vi "Init.vi"(4 "Virt Instrs":string="{\n\t\"Virt Instrs\": [\n\t\t{\"Target Ident\": \"Photosensor\",\"Instr Ident\": \"SimulatedScope\",\"Const Action Data\": \"0\",\"Class\": \"HAL GOOP4.lvlib:Virt Instr Base.lvclass\"},\n\t\t{\"Target Ident\": \"Powersensor\",\"Instr Ident\": \"SimulatedScope\",\"Const Action Data\": \"1\",\"Class\": \"Virt Instrs Scope.lvlib:Virt Voltage Reader.lvclass\"},\n\t\t{\"Target Ident\": \"Excitation\",\"Instr Ident\": \"SimulatedFGen\",\"Const Action Data\": \"0\",\"Class\": \"Virt Instrs FGen.lvlib:Virt Voltage Generator.lvclass\"}\n\t]\n}", 6 "Instr CFGs":string[](array[string]), 8 "error in (no error)":errorcluster, 11 "HAL GOOP4:Series Base in":refnum<class "Series Base.lvclass">) -> (0 "error out":errorcluster, 3 "HAL GOOP4:Series Base out":refnum<class "Series Base.lvclass">)   [LabVIEW 2023, in "HAL GOOP4.lvlib" / "Series Base.lvclass"]
uses:
  Series Base.lvclass
  Series Base.lvclass/Series Base.ctl
  Measure and Stimulus Subsystems/Measure and Stimulus Subsystems.lvclass
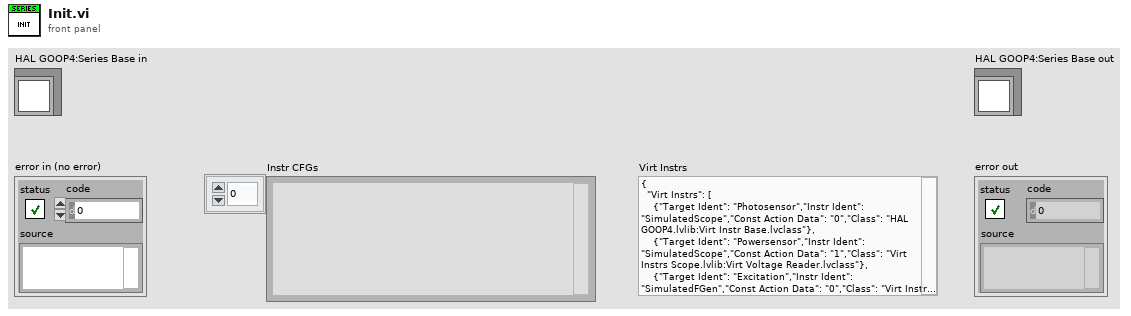
[diagram p1: front panel]
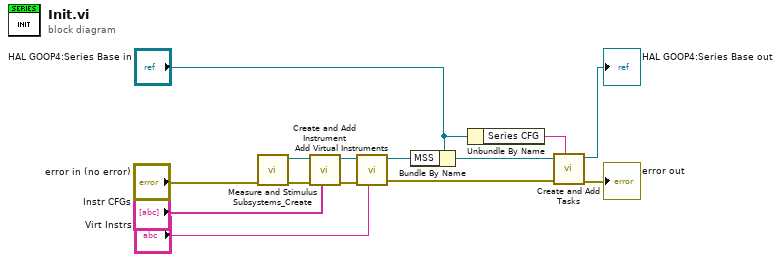
[diagram p0: block diagram]
diagram:
  n1 = call "Measure and Stimulus Subsystems_Create.vi"("Error In"="error in (no error)") -> ("Error Out"=w14:errorcluster, "reference out"=w12:refnum<class "Measure and Stimulus Subsystems.lvclass">)  [unwired: 9 in]
  n2 = call "Create and Add Instrument.vi"("Physical Intr Configs"="Instr CFGs", "Error In"=w14, "reference in"=w12) -> ("Error Out"=w13:errorcluster, "reference out"=w11:refnum<class "Measure and Stimulus Subsystems.lvclass">)  [unwired: 7 in]
  n3 = call "Add Virtual Instruments.vi"("<JSON CFG>"="Virt Instrs", "Error In"=w13, "reference in"=w11) -> ("Error Out"=w8:errorcluster, "reference out"=w4:refnum<class "Measure and Stimulus Subsystems.lvclass">)  [unwired: 7 in]
  n4 = Bundle By Name(cluster="HAL GOOP4:Series Base in", "MSS"=w4) -> (w3:refnum<class "Series Base.lvclass">)
  n5 = Unbundle By Name("HAL GOOP4:Series Base in") -> ("Series CFG"=w6:string)
  n6 = call-dynamic "Create and Add Tasks.vi"("Tasks <JSON>"=w6, "error in (no error)"=w8, "HAL GOOP4:Series Base in"=w3) -> ("error out"=→"error out":errorcluster, "HAL GOOP4:Series Base out"=→"HAL GOOP4:Series Base out":refnum<class "Series Base.lvclass">)  [unwired: 7 in]
